vi "Init UI Refs.vi"(8 "error in (no error)":errorcluster, 11 "HistorianCharting in":refnum<class "HistorianCharting.lvclass">) -> (0 "error out":errorcluster, 3 "HistorianCharting out":refnum<class "HistorianCharting.lvclass">)   [LabVIEW 2020, in "VolatusGUIElements.lvlib" / "HistorianCharting.lvclass"]
uses:
  HistorianCharting.lvclass
  C:/dev/lv20CE/relink/lv-volatus/VolatusGUI/GUI Element/GUI Element.lvclass
  VolatusGUI/GUI Element/GUI Element.lvclass/GUI Element.ctl
  HistorianCharting.lvclass/HistorianCharting.ctl
  VolatusGUI/GUI Element/GUI Element.lvclass
  C:/dev/lv20CE/relink/lv-volatus/VolatusGUIElements/HistorianCharting/HistorianCharting.lvclass
  C:/dev/lv20CE/relink/lv-volatus/VolatusGUI/OnValueChangeHandler/OnValueChangeHandler.lvclass
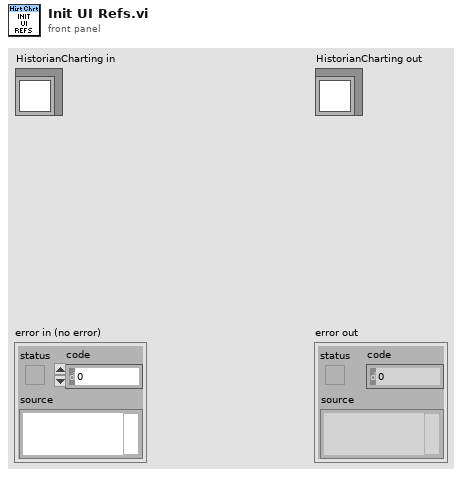
[diagram p1: front panel]
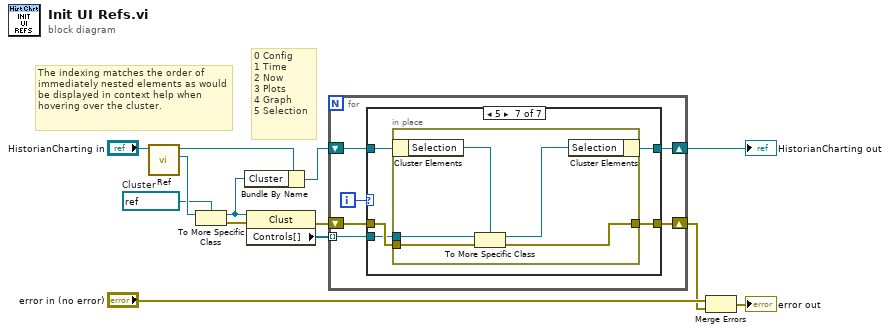
[diagram p0: block diagram]
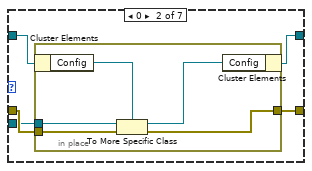
[diagram p3: hidden frame]
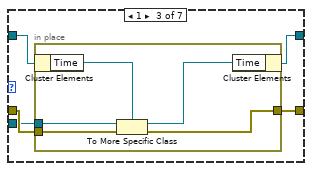
[diagram p4: hidden frame]
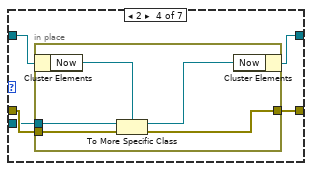
[diagram p5: hidden frame]
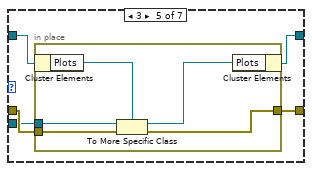
[diagram p6: hidden frame]
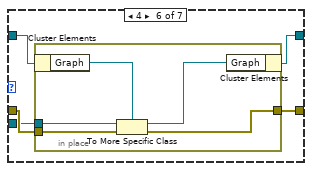
[diagram p7: hidden frame]
diagram:
  w10 = refnum<vi> refnum  # Cluster
  # "The indexing matches the order of immediately nested elements as would be displayed in context help when hovering over the cluster."
  # "0 Config\n1 Time\n2 Now\n3 Plots\n4 Graph\n5 Selection"
  n1 = call "Ref.vi"("GUI Element in"="HistorianCharting in") -> ("Ref"=w11:refnum<vi>, "GUI Element out"=w8:refnum<class "HistorianCharting.lvclass">)  [unwired: 9 in]
  n2 = To More Specific Class(target class=w10, reference=w11) -> (specific class reference=w1:refnum<vi>, error out=w9:errorcluster)  [unwired: 1 in]
  n3 = Bundle By Name(cluster=w8, "Cluster"=w1) -> (w2:refnum<class "HistorianCharting.lvclass">)
  n4 = property class="Clust"(reference=w1, error in=w9) -> (error out=w6:errorcluster, "Controls[]"=w7:refnum<vi>[])  [unwired: 1 out]
  n5 = for {
    shift-right: [w15] -> w5
    shift-left: w2 -> [w17]
    tunnel: w7 -> [w16] mode=indexing
    shift-right: [w14] -> w3
    shift-left: w6 -> [w18]
    i -> [w19]
    n6 = case shown="5" w19 {
      tunnel: w18 -> [w20 w26 w36 w46 w56 w66 w76]
      tunnel: w17 -> [w21 w23 w33 w43 w53 w63 w73]
      tunnel: w16 -> [_ w25 w35 w45 w55 w65 w75]
      tunnel: [w21 w22 w32 w42 w52 w62 w72] -> w15
      tunnel: [w20 w24 w34 w44 w54 w64 w74] -> w14
      frame Default {
      }
      frame 0 {
        n7 = in-place {
          in-place-border: w26 -> [w31]
          in-place-border: w25 -> [w30]
          in-place-border: [w29] -> w24
          n8 = in-place-cluster #1(w23) -> ("Config"=w28:refnum<vi>)
          n9 = To More Specific Class(target class=w28, reference=w30, error in=w31) -> (specific class reference=w27:refnum<vi>, error out=w29:errorcluster)
          n10 = in-place-cluster #1("Config"=w27) -> (w22:refnum<class "HistorianCharting.lvclass">)
        }
      }
      frame 1 {
        n11 = in-place {
          in-place-border: w36 -> [w41]
          in-place-border: w35 -> [w40]
          in-place-border: [w39] -> w34
          n12 = in-place-cluster #2(w33) -> ("Time"=w38:refnum<vi>)
          n13 = To More Specific Class(target class=w38, reference=w40, error in=w41) -> (specific class reference=w37:refnum<vi>, error out=w39:errorcluster)
          n14 = in-place-cluster #2("Time"=w37) -> (w32:refnum<class "HistorianCharting.lvclass">)
        }
      }
      frame 2 {
        n15 = in-place {
          in-place-border: w46 -> [w51]
          in-place-border: w45 -> [w50]
          in-place-border: [w49] -> w44
          n16 = in-place-cluster #3(w43) -> ("Now"=w48:refnum<vi>)
          n17 = To More Specific Class(target class=w48, reference=w50, error in=w51) -> (specific class reference=w47:refnum<vi>, error out=w49:errorcluster)
          n18 = in-place-cluster #3("Now"=w47) -> (w42:refnum<class "HistorianCharting.lvclass">)
        }
      }
      frame 3 {
        n19 = in-place {
          in-place-border: w56 -> [w61]
          in-place-border: w55 -> [w60]
          in-place-border: [w59] -> w54
          n20 = in-place-cluster #4(w53) -> ("Plots"=w58:refnum<vi>)
          n21 = To More Specific Class(target class=w58, reference=w60, error in=w61) -> (specific class reference=w57:refnum<vi>, error out=w59:errorcluster)
          n22 = in-place-cluster #4("Plots"=w57) -> (w52:refnum<class "HistorianCharting.lvclass">)
        }
      }
      frame 4 {
        n23 = in-place {
          in-place-border: w66 -> [w71]
          in-place-border: w65 -> [w70]
          in-place-border: [w69] -> w64
          n24 = in-place-cluster #5(w63) -> ("Graph"=w68:refnum<vi>)
          n25 = To More Specific Class(target class=w68, reference=w70, error in=w71) -> (specific class reference=w67:refnum<vi>, error out=w69:errorcluster)
          n26 = in-place-cluster #5("Graph"=w67) -> (w62:refnum<class "HistorianCharting.lvclass">)
        }
      }
      frame 5 {
        n27 = in-place {
          in-place-border: w76 -> [w81]
          in-place-border: w75 -> [w80]
          in-place-border: [w79] -> w74
          n28 = in-place-cluster #6(w73) -> ("Selection"=w78:refnum<vi>)
          n29 = To More Specific Class(target class=w78, reference=w80, error in=w81) -> (specific class reference=w77:refnum<vi>, error out=w79:errorcluster)
          n30 = in-place-cluster #6("Selection"=w77) -> (w72:refnum<class "HistorianCharting.lvclass">)
        }
      }
    }
  }
  "HistorianCharting out" <- w5
  n31 = Merge Errors("error in (no error)", w3) -> (→"error out":errorcluster)
